vi "Write State Name.vi"(8 "error in (no error)":errorcluster, 10 "State Name":string, 11 "Command State Actor in":refnum<class "Command State Actor.lvclass">) -> (0 "error out":errorcluster, 3 "Command State Actor out":refnum<class "Command State Actor.lvclass">)   [LabVIEW 2013, in "Command State Actor.lvlib" / "Command State Actor.lvclass"]
uses:
  Command State Actor.lvclass
  Command State Actor.lvclass/Command State Actor.ctl
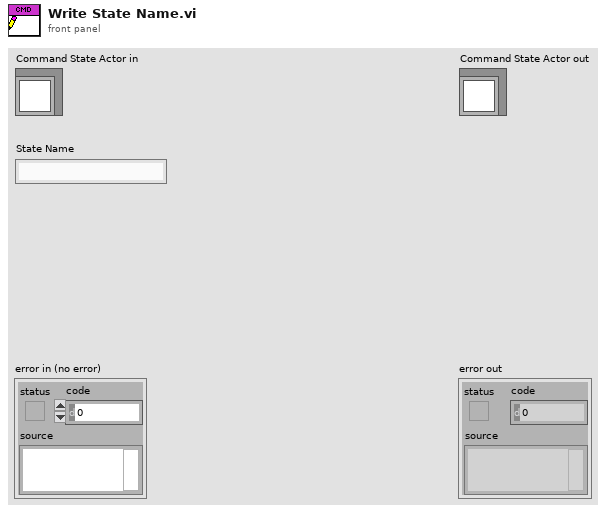
[diagram p1: front panel]
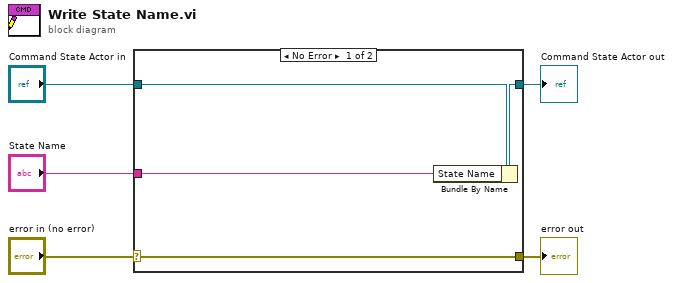
[diagram p0: block diagram]
diagram:
  n1 = case shown="No Error" "error in (no error)" {
    selector: "error in (no error)" -> [w9 w10]
    tunnel: [w9 w10] -> w4
    tunnel: [w7 w11] -> w2
    tunnel: "Command State Actor in" -> [w8 w11]
    tunnel: "State Name" -> [w6 _]
    frame No Error {
      n2 = Bundle By Name(cluster=w8, "State Name"=w6) -> (w7:refnum<class "Command State Actor.lvclass">)
    }
    frame Error {
    }
  }
  "error out" <- w4
  "Command State Actor out" <- w2
